vi "Drive Tasks.vi"(1 "Drive Parameters":T1) -> ()   [LabVIEW 2015]
uses:
  <vilib>/Rock Robotics/WPI/Utilities/WPI_GetSetVariantRefNum.vi
  Robot Global Data.vi
  <vilib>/Rock Robotics/WPI/RobotDrive/WPI_RobotDriveArcadeDrive_Standard(NoSaturation).vi
  <vilib>/Rock Robotics/Network Tables/NT Write Numeric Array.vi
panel:
  out "Centered Time":i32(graph)
  out "Gyro Rate":dbl
  out "Drive Operation":enum16{"Turn Robot", "Drive Straight for Time"}(ring)
  out "Set Point":dbl
  out "Current Gyro Value":dbl
  out "Iteration":i32
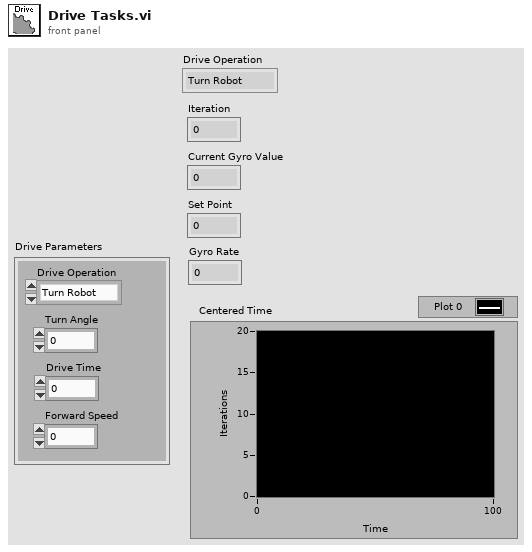
[diagram p1: front panel]
types:
  T1 = cluster{"Drive Operation":enum16{"Turn Robot", "Drive Straight for Time"}, "Turn Angle":dbl, "Drive Time":dbl, "Forward Speed":dbl}
  T2 = typedef "WPI_GyroDevRef.ctl" = cluster{"DevStatus":errorcluster, "Analog Channel":T3, "Offset":dbl, "Gain (VoltsPerDegree/Second)":dbl, "Gyro Type":enum16{"Analog", "XRS450"}, "Handle":i32, "SPI Bus":T4, "Device Found":bool, "Sample Rate":dbl, "Calibrate On Open":bool}
  T3 = typedef "FPGA_AIChannel.ctl" = enum8{"AI 0", "AI 1", "AI 2", "AI 3", "AI MXP 0", "AI MXP 1", "AI MXP 2", "AI MXP 3", "Invalid"}
  T4 = typedef "spi_bus.ctl" = enum16{"SPI On-Board, CS0", "SPI On-Board, CS1", "SPI On-Board, CS2", "SPI On-Board, CS3", "SPI MXP", "Invalid"}
  T5 = typedef "WPI_RobotDriveDevRef.ctl" = cluster{"DevStatus":errorcluster, "Motors[]":T6[], "Square Inputs":bool, "Max Output":dbl}
  T6 = typedef "WPI_MotorControlDeviceRef.ctl" = cluster{"DeviceStatus":errorcluster, "Type":T7, "PWM":cluster{"PWM Channel":T8, "DeadBand":T9}, "CAN":cluster{"Device Number":u8, "Control Mode":T10, "Semaphore":T11, "Max Vout":dbl, "TalonSRX Control Mode":T12}, "Invert":bool}
  T7 = typedef "WPI_MotorControlType.ctl" = enum16{"PWM", "CAN", "CANTalonSRX"}
  T8 = typedef "FPGA_DIOPWMChannel.ctl" = enum8{"PWM 0", "PWM 1", "PWM 2", "PWM 3", "PWM 4", "PWM 5", "PWM 6", "PWM 7", "PWM 8", "PWM 9", "PWM MXP 0", "PWM MXP 1", "PWM MXP 2", "PWM MXP 3", "PWM MXP 4", "PWM MXP 5", "PWM MXP 6", "PWM MXP 7", "PWM MXP 8", "PWM MXP 9", "Invalid"}
  T9 = typedef "WPI_PWMDeadband.ctl" = cluster{"Name":string, "maxPositivePwm":i32, "minPositivePwm":i32, "centerPwm":i32, "maxNegativePwm":i32, "minNegativePwm":i32, "angularRange":u16}
  T10 = typedef "WPI_CANJaguar_ControlMode.ctl" = enum8{"Percent VBus", "Current", "Speed", "Position", "Voltage"}
  T11 = typedef "Semaphore RefNum" = refnum<k1>
  T12 = typedef "WPI_CANTalonSRX_APIControlMode.ctl" = enum8{"Percent VBus", "Speed", "Position", "Slave", "Unchanged / Invalid", "Voltage Compensation", "Current", "Motion Profile"}
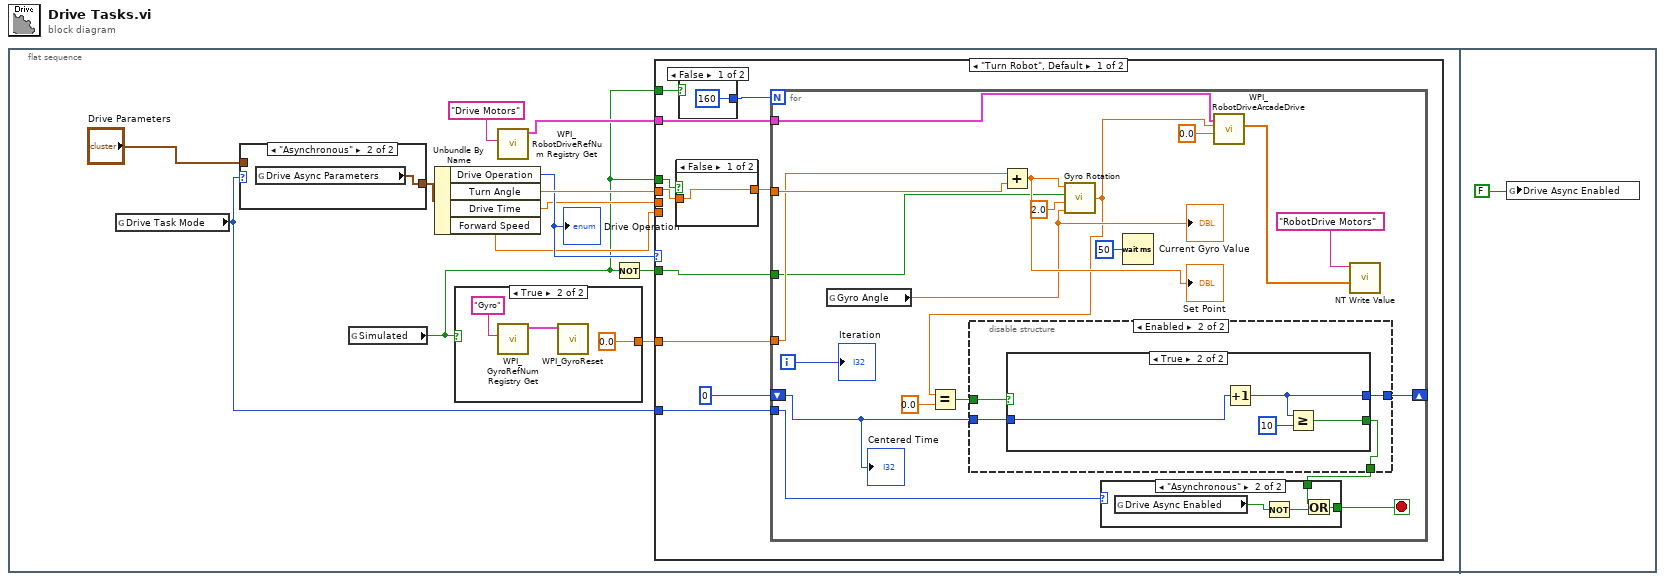
[diagram p0: block diagram]
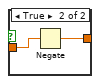
[diagram p2: hidden frame]
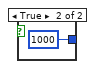
[diagram p3: hidden frame]
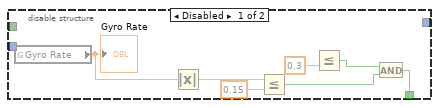
[diagram p4: hidden frame]
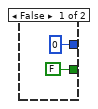
[diagram p5: hidden frame]
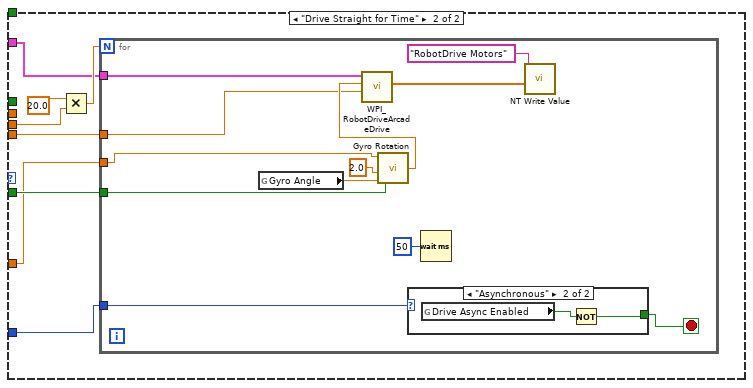
[diagram p7: hidden frame]
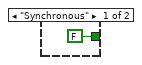
[diagram p8: hidden frame]
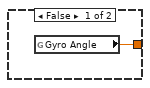
[diagram p9: hidden frame]
diagram:
  n1 = flat-sequence {
    frame #0 {
      n2 = global read "Robot Global Data.vi" "Drive Task Mode"() -> (w7:enum16{"Synchronous", "Asynchronous"})
      n3 = case shown="\"Asynchronous\"" w7 {
        tunnel: [w98 w99] -> w10
        tunnel: "Drive Parameters" -> [w98 _]
        frame "Synchronous" {
        }
        frame "Asynchronous" {
          n4 = global read "Robot Global Data.vi" "Drive Async Parameters"() -> (w99:T1)
        }
      }
      n5 = global read "Robot Global Data.vi" "Simulated"() -> (w1:bool)
      n6 = Unbundle By Name(w10) -> ("Drive Operation"=w4:enum16{"Turn Robot", "Drive Straight for Time"}, "Turn Angle"=w9:dbl, "Drive Time"=w3:dbl, "Forward Speed"=w2:dbl)
      "Drive Operation" <- w4
      n7 = case shown="True" w1 {
        tunnel: [w94 0.0 ("Gyro Angle")] -> w6
        frame False {
          n8 = global read "Robot Global Data.vi" "Gyro Angle"() -> (w94:dbl)
        }
        frame True {
          n9 = call <vilib>:"WPI_GyroRefNum Registry Get.vi"("refnum name"="Gyro") -> ("GyroDevRef"=w96:T2)  [unwired: 9 in, 1 out]
          n10 = call <vilib>:"WPI_GyroReset.vi"("GyroDevRef"=w96) -> ()  [unwired: 9 in, 2 out]
        }
      }
      n11 = call <vilib>:"WPI_RobotDriveRefNum Registry Get.vi"("refnum name"="Drive Motors") -> ("RobotDriveDevRef"=w11:T5)  [unwired: 1 in, 9 out]
      n12 = Not(x=w1) -> (.not. x?=w5:bool)
      n13 = case shown="\"Turn Robot\", Default" w4 {
        tunnel: w11 -> [w21 w72]
        tunnel: w9 -> [w14 _]
        tunnel: w7 -> [w20 w78]
        tunnel: w6 -> [w19 w73]
        tunnel: w5 -> [w18 w74]
        tunnel: w3 -> [_ w77]
        tunnel: w2 -> [_ w71]
        tunnel: w1 -> [w16 _]
        tunnel: w1 -> [w15 _]
        frame "Turn Robot", Default {
          n14 = case shown="False" w15 {
            tunnel: w14 -> [w23 w25]
            tunnel: [w23 w24] -> w13
            frame False {
            }
            frame True {
              n15 = Negate(x=w25) -> (-x=w24:dbl)
            }
          }
          n16 = case shown="False" w16 {
            tunnel: [160 1000] -> w22
            frame False {
            }
            frame True {
            }
          }
          n17 = for {
            N: w22 -> [_]
            tunnel: w21 -> [w46]
            tunnel: w13 -> [w41]
            tunnel: w19 -> [w39]
            tunnel: w20 -> [w35]
            tunnel: w18 -> [w34]
            shift-right: [w29] -> _
            shift-left: 0 -> [w28]
            i -> [w43]
            stop <- w38 stop-if-true
            n18 = global read "Robot Global Data.vi" "Gyro Angle"() -> (w40:dbl)
            "Current Gyro Value" <- w40
            n19 = Add(x=w39, y=w41) -> (x+y=w44:dbl)
            "Set Point" <- w44
            n20 = call "Gyro Rotation.vi"("Current Value"=w40, "Deadband"=2.0, "Invert Rotation"=w34, "Set Point"=w44) -> ("Rotation"=w31:dbl)
            n21 = Equal?(x=w31, y=0.0) -> (x = y?=w30:bool)
            n22 = disable-structure shown="Enabled" {
              disable-tunnel: [w49 w56] -> w33
              disable-tunnel: w30 -> [_ w59]
              disable-tunnel: [_ w58] -> w29
              disable-tunnel: w28 -> [_ w57]
              frame Disabled {
                n23 = global read "Robot Global Data.vi" "Gyro Rate"() -> (w54:dbl)
                "Gyro Rate" <- w54
                n24 = Absolute Value(x=w54) -> (abs(x)=w53:dbl)
                n25 = Less Or Equal?(x=w53, y=0.15) -> (x <= y?=w51:bool)
                n26 = Less Or Equal?(y=0.3) -> (x=w48:dbl, x <= y?=w50:bool)
                n27 = And(x=w50, y=w51) -> (x .and. y?=w49:bool)
              }
              frame Enabled {
                n28 = case shown="True" w59 {
                  tunnel: [0 w64] -> w58
                  tunnel: w57 -> [_ w65]
                  tunnel: [FALSE w62] -> w56
                  frame False {
                  }
                  frame True {
                    n29 = Increment(x=w65) -> (x+1=w64:i32)
                    n30 = Greater Or Equal?(x=w64, y=10) -> (x >= y?=w62:bool)
                  }
                }
              }
            }
            n31 = case shown="\"Asynchronous\"" w35 {
              tunnel: [w66 w70] -> w38
              tunnel: w33 -> [w66 w69]
              frame "Synchronous" {
              }
              frame "Asynchronous" {
                n32 = global read "Robot Global Data.vi" "Drive Async Enabled"() -> (w68:bool)
                n33 = Not(x=w68) -> (.not. x?=w67:bool)
                n34 = Or(x=w69, y=w67) -> (x .or. y?=w70:bool)
              }
            }
            n35 = Wait (ms)(milliseconds to wait=u32 50) -> ()  [unwired: 1 out]
            n36 = call-poly <vilib>:"WPI_RobotDriveArcadeDrive.vi"("Y axis value"=0.0, "X axis value"=w31, "RobotDriveDevRef"=w46) -> ("Motor Values"=w36:dbl[])  [unwired: 6 in, 2 out]
            n37 = call-poly <vilib>:"NT Write Value.vi"("Numeric Array"=w36, "Name"="RobotDrive Motors") -> ()  [unwired: 9 in, 1 out]
            "Iteration" <- w43
            "Centered Time" <- w28
          }
        }
        frame "Drive Straight for Time" {
          n38 = Multiply(x=20.0, y=w77) -> (x*y=w75:dbl)
          n39 = for {
            N: w75 -> [_]
            tunnel: w78 -> [w90]
            tunnel: w74 -> [w87]
            tunnel: w73 -> [w85]
            tunnel: w72 -> [w83]
            tunnel: w71 -> [w79]
            stop <- w89 stop-if-true
            n40 = global read "Robot Global Data.vi" "Gyro Angle"() -> (w84:dbl)
            n41 = call "Gyro Rotation.vi"("Current Value"=w84, "Deadband"=2.0, "Invert Rotation"=w87, "Set Point"=w85) -> ("Rotation"=w82:dbl)
            n42 = call-poly <vilib>:"WPI_RobotDriveArcadeDrive.vi"("Y axis value"=w79, "X axis value"=w82, "RobotDriveDevRef"=w83) -> ("Motor Values"=w81:dbl[])  [unwired: 6 in, 2 out]
            n43 = case shown="\"Asynchronous\"" w90 {
              tunnel: [FALSE w92] -> w89
              frame "Synchronous" {
              }
              frame "Asynchronous" {
                n44 = global read "Robot Global Data.vi" "Drive Async Enabled"() -> (w93:bool)
                n45 = Not(x=w93) -> (.not. x?=w92:bool)
              }
            }
            n46 = Wait (ms)(milliseconds to wait=u32 50) -> ()  [unwired: 1 out]
            n47 = call-poly <vilib>:"NT Write Value.vi"("Numeric Array"=w81, "Name"="RobotDrive Motors") -> ()  [unwired: 9 in, 1 out]
          }
        }
      }
    }
    frame #1 {
      n48 = global write "Robot Global Data.vi" "Drive Async Enabled"(FALSE) -> ()
    }
  }
